vi "CallBack Key Value.vi"(6 "Variant":variant, 8 "error in (no error)":errorcluster, 9 "Old Values":string[][](array[string]), 10 "object ref in":T1, 11 "Table Change":T2) -> (0 "error out":errorcluster)   [LabVIEW 2013, in "control module editor.lvclass"]
uses:
  control module editor.lvclass
  Table API/Table Manager/Cell Change.ctl
  Table API/Table Manager/object ref.ctl
  Configuration Editor/Classes/Engine Parent/Engine Parent Editor Node.lvclass
  Configuration Editor/Classes/Module editor node/module editor node.lvclass
  configuration/control module configuration.lvclass
  read fixed channel configuration.vi
  Table API/Table Manager.lvlib
  Table API/Table Manager/Table Manager.lvclass
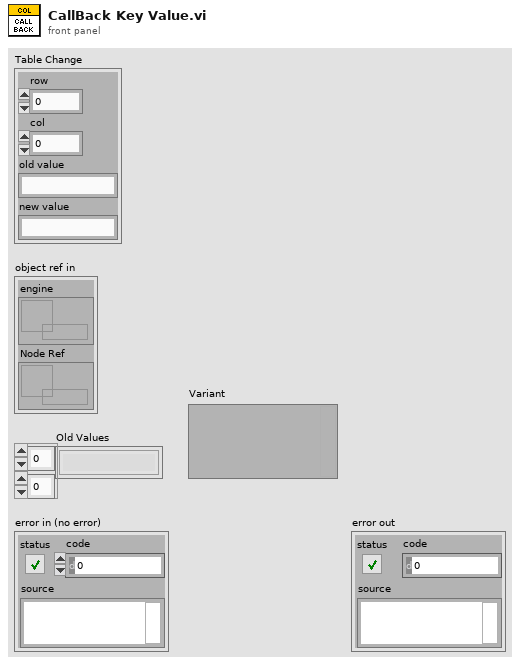
[diagram p1: front panel]
types:
  T1 = typedef "Table Manager.lvlib/Table Manager.lvclass/object ref.ctl" = cluster{"engine":refnum<data-value>, "Node Ref":refnum<data-value>}
  T2 = typedef "Table Manager.lvlib/Cell Change.ctl" = cluster{"row":i32, "col":i32, "old value":string, "new value":string}
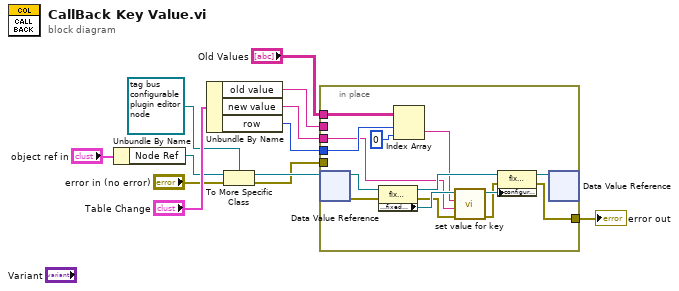
[diagram p0: block diagram]
diagram:
  n1 = Unbundle By Name("object ref in") -> ("Node Ref"=w4:refnum<data-value>)
  n2 = Unbundle By Name("Table Change") -> ("old value"=w12:string, "new value"=w11:string, "row"=w6:i32)
  n3 = To More Specific Class(target class=refnum<data-value> refnum ("data value reference"), reference=w4, error in="error in (no error)") -> (specific class reference=w3:refnum<data-value>, error out=w1:errorcluster)
  n4 = in-place {
    in-place-border: [w18] -> w10
    in-place-border: w1 -> [_]
    in-place-border: w12 -> [_]
    in-place-border: w11 -> [w13]
    in-place-border: "Old Values" -> [w26]
    in-place-border: w6 -> [w25]
    n5 = in-place-dvr #1(w3) -> (w24:refnum<class "control module editor.lvclass">, w16:errorcluster)
    n6 = property class="fixed channel editor node"(reference=w24, error in=w16) -> (reference out=w21:refnum<class "control module editor.lvclass">, error out=w17:errorcluster, "Properties:fixed channel configuration"=w23:refnum<class "control module configuration.lvclass">)
    n7 = Index Array(array=w26, index (row)=w25, index (col)=0 ("disabled index (col)")) -> (element=w14:string)
    n8 = call-dynamic "set value for key.vi"("error in"=w17, "value"=w13, "key"=w14, "fixed channel configuration in"=w23) -> ("error out"=w19:errorcluster, "fixed channel configuration out"=w22:refnum<class "control module configuration.lvclass">)  [unwired: 6 in]
    n9 = property class="fixed channel editor node"(reference=w21, error in=w19, "configuration"=w22) -> (reference out=w20:refnum<class "control module editor.lvclass">, error out=w18:errorcluster)
    n10 = in-place-dvr #1(w20) -> ()  [unwired: 2 out]
  }
  "error out" <- w10
